vi "AutoAction.vi"(8 "Shoot Percentage":i32, 10 "Case":string) -> ()   [LabVIEW 2016]
uses:
  <vilib>/Rock Robotics/WPI/Utilities/WPI_GetSetVariantRefNum.vi
  <vilib>/Rock Robotics/WPI/RobotDrive/WPI_RobotDriveMecanumDrive_Cartesian.vi
  Robot Global Data.vi
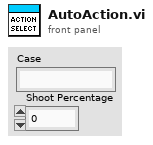
[diagram p1: front panel]
types:
  T1 = typedef "WPI_SwitchDevRef.ctl" = cluster{"DevStatus":errorcluster, "DIO Channel":T2, "CntIndex":T3, "Normally Closed":bool}
  T2 = typedef "FPGA_DIOChannel.ctl" = enum8{"DIO 0", "DIO 1", "DIO 2", "DIO 3", "DIO 4", "DIO 5", "DIO 6", "DIO 7", "DIO 8", "DIO 9", "DIO MXP 0", "DIO MXP 1", "DIO MXP 2", "DIO MXP 3", "DIO MXP 4", "DIO MXP 5", "DIO MXP 6", "DIO MXP 7", "DIO MXP 8", "DIO MXP 9", "DIO MXP 10", "DIO MXP 11", "DIO MXP 12", "DIO MXP 13", "DIO MXP 14", "DIO MXP 15", "SPI Port CS1", "SPI Port CS2", "SPI Port CS3", "SPI Port MISO", "SPI Port MOSI", "Invalid"}
  T3 = typedef "FPGA_CounterCtrSystemIndex.ctl" = enum8{"Ctr 0", "Ctr 1", "Ctr 2", "Ctr 3", "Ctr 4", "Ctr 5", "Ctr 6", "Ctr 7", "Invalid"}
  T4 = typedef "WPI_RobotDriveDevRef.ctl" = cluster{"DevStatus":errorcluster, "Motors[]":T5[], "Square Inputs":bool, "Max Output":dbl}
  T5 = typedef "WPI_MotorControlDeviceRef.ctl" = cluster{"DeviceStatus":errorcluster, "Type":T6, "PWM":cluster{"PWM Channel":T7, "DeadBand":T8}, "CAN":cluster{"Device Number":u8, "SetOutput VI Ref":variant, "GetOutput VI Ref":variant, "Enable VI Ref":variant, "Disable VI Ref":variant, "Data":variant}, "Invert":bool}
  T6 = typedef "WPI_MotorControlType.ctl" = enum16{"PWM", "CAN"}
  T7 = typedef "FPGA_DIOPWMChannel.ctl" = enum8{"PWM 0", "PWM 1", "PWM 2", "PWM 3", "PWM 4", "PWM 5", "PWM 6", "PWM 7", "PWM 8", "PWM 9", "PWM MXP 0", "PWM MXP 1", "PWM MXP 2", "PWM MXP 3", "PWM MXP 4", "PWM MXP 5", "PWM MXP 6", "PWM MXP 7", "PWM MXP 8", "PWM MXP 9", "Invalid"}
  T8 = typedef "WPI_PWMDeadband.ctl" = cluster{"Name":string, "maxPositivePwm":i32, "minPositivePwm":i32, "centerPwm":i32, "maxNegativePwm":i32, "minNegativePwm":i32, "angularRange":u16}
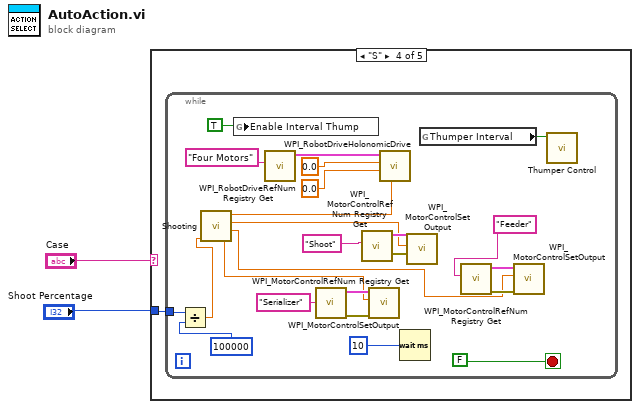
[diagram p0: block diagram]
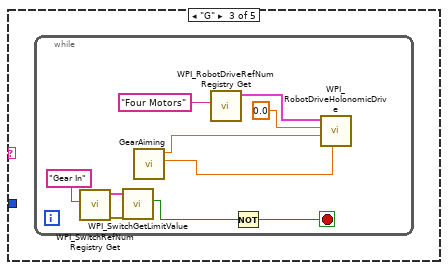
[diagram p4: hidden frame]
diagram:
  n1 = case shown="\"S\"" "Case" {
    tunnel: "Shoot Percentage" -> [_ _ _ w13 _]
    frame "N", Default {
    }
    frame "C" {
    }
    frame "G" {
      n2 = while {
        stop <- w4 stop-if-true
        n3 = call <vilib>:"WPI_SwitchRefNum Registry Get.vi"("refnum name"="Gear In") -> ("error out"=w7:errorcluster, "SwitchDevRef"=w6:T1)  [unwired: 9 in]
        n4 = call <vilib>:"WPI_SwitchGetLimitValue.vi"("error in (no error)"=w7, "SwitchDevRef"=w6) -> ("Switch Pressed"=w5:bool)  [unwired: 7 in, 2 out]
        n5 = call "GearAiming.vi"() -> ("Drive Rotate"=w9:dbl, "Drive Y"=w8:dbl)  [unwired: 10 in]
        n6 = call <vilib>:"WPI_RobotDriveRefNum Registry Get.vi"("refnum name"="Four Motors") -> ("RobotDriveDevRef"=w12:T4)  [unwired: 9 in, 1 out]
        n7 = Not(x=w5) -> (.not. x?=w4:bool)
        n8 = call-poly <vilib>:"WPI_RobotDriveHolonomicDrive.vi"("Rotation"=w9, "Y"=w8, "X"=0.0, "RobotDriveDevRef"=w12) -> ()  [unwired: 5 in, 3 out]
      }
    }
    frame "S" {
      n9 = while {
        tunnel: w13 -> [w22]
        stop <- FALSE stop-if-true
        n10 = Divide(x=w22, y=100000) -> (x/y=w21:dbl)
        n11 = call "Shooting.vi"("Shoot override"=w21) -> ("Serializer Output"=w25:dbl, "Feeder Output"=w16:dbl, "Shooter \nPWM"=w34:dbl, "Rotation Out"=w29:dbl)  [unwired: 5 in]
        n12 = global write "Robot Global Data.vi" "Enable Interval Thump"(TRUE ("Thumper Out")) -> ()
        n13 = call <vilib>:"WPI_RobotDriveRefNum Registry Get.vi"("refnum name"="Four Motors") -> ("RobotDriveDevRef"=w33:T4)  [unwired: 9 in, 1 out]
        n14 = call <vilib>:"WPI_MotorControlRefNum Registry Get.vi"("refnum name"="Serializer") -> ("error out"=w28:errorcluster, "MotorControlDevRef"=w27:T5)  [unwired: 9 in]
        n15 = call <vilib>:"WPI_MotorControlRefNum Registry Get.vi"("refnum name"="Shoot") -> ("error out"=w36:errorcluster, "MotorControlDevRef"=w35:T5)  [unwired: 9 in]
        n16 = call <vilib>:"WPI_MotorControlSetOutput.vi"("error in (no error)"=w28, "Output"=w25, "MotorControlDevRef"=w27) -> ()  [unwired: 6 in, 3 out]
        n17 = call-poly <vilib>:"WPI_RobotDriveHolonomicDrive.vi"("Rotation"=w29, "Y"=0.0, "X"=0.0, "RobotDriveDevRef"=w33) -> ()  [unwired: 5 in, 3 out]
        n18 = Wait (ms)(milliseconds to wait=10) -> ()  [unwired: 1 out]
        n19 = call <vilib>:"WPI_MotorControlSetOutput.vi"("error in (no error)"=w36, "Output"=w34, "MotorControlDevRef"=w35) -> ()  [unwired: 6 in, 3 out]
        n20 = global read "Robot Global Data.vi" "Thumper Interval"() -> (w18:bool)
        n21 = call <vilib>:"WPI_MotorControlRefNum Registry Get.vi"("refnum name"="Feeder") -> ("error out"=w17:errorcluster, "MotorControlDevRef"=w14:T5)  [unwired: 9 in]
        n22 = call <vilib>:"WPI_MotorControlSetOutput.vi"("error in (no error)"=w17, "Output"=w16, "MotorControlDevRef"=w14) -> ()  [unwired: 6 in, 3 out]
        n23 = call "Thumper Control.vi"("Thump"=w18) -> ()  [unwired: 11 in]
      }
    }
    frame "H" {
    }
  }
